vi "Get User Interface Information.vi"(8 "error in (no error)":errorcluster, 11 "measurement plugin in":refnum<class "Example Plugin.lvclass">) -> (0 "error out":errorcluster, 2 "user interface information":T1[](array[typedef]), 3 "measurement plugin out":refnum<class "Example Plugin.lvclass">)   [LabVIEW 2025, in "Example Plugin.lvclass"]
uses:
  Example Plugin.lvclass
  <vilib>/Plug-In SDKs/Measurements/Helpers/TypeDefs/User Interface Information.ctl
  Example Plugin.lvclass/Example Plugin.ctl
  <vilib>/Plug-In SDKs/Measurements/NI Measurement Plug-In SDK.lvlib
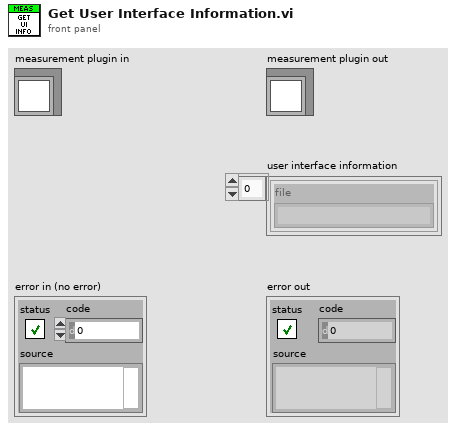
[diagram p1: front panel]
types:
  T1 = typedef "NI Measurement Plug-In SDK.lvlib/User Interface Information.ctl" = cluster{"file":string}
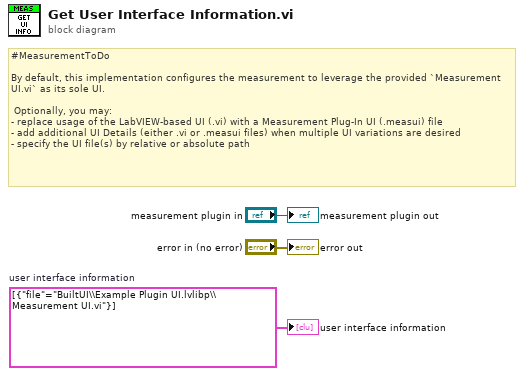
[diagram p0: block diagram]
diagram:
  w1 = T1[] [{"file"="BuiltUI\\Example Plugin UI.lvlibp\\Measurement UI.vi"}]  # user interface information
  # "#MeasurementToDo\n\nBy default, this implementation configures the measurement to leverage the provided `Measurement UI.vi` as its sole UI.\n\n Optionally, you may:\n- replace usage of the LabVIEW-based UI (.vi) with a Measurement Plug-In UI (.measui) file\n- add additional UI Details (either .vi or .measui files) when multiple UI variations are desired\n- specify the UI file(s) by relative or absolute path"
  "error out" <- "error in (no error)"
  "measurement plugin out" <- "measurement plugin in"
  "user interface information" <- w1
